vi "Get JTAG Scan Chain IDCODEs.vi"(8 "Error In":errorcluster, 11 "Adept Device":T1) -> (0 "Error In":errorcluster, 2 "IDCODEs":u32[](array[numeric]), 3 "Adept Device":T1)   [LabVIEW 2011, in "LVH-Adept.lvlib"]
doc: "Get the JTAG Scan Chain IDCODEs from a Digilent FPGA board."
uses:
  <vilib>/LabVIEW Hacker/Adept/LVH-Adept.lvlib
  Private/Type Defs/Device Config.ctl
  Private/Type Defs/Status.ctl
  Private/DJTG/DJTG.lvlib
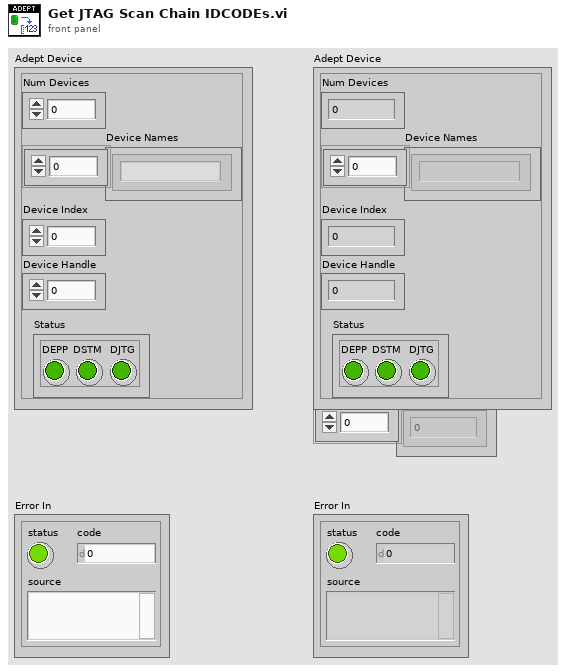
[diagram p1: front panel]
types:
  T1 = typedef "LVH-Adept.lvlib/Device Config.ctl" = cluster{"Num Devices":i32, "Device Names":string[], "Device Index":u16, "Device Handle":u32, "Status":T2}
  T2 = typedef "LVH-Adept.lvlib/Status.ctl" = cluster{"DEPP":bool, "DSTM":bool, "DJTG":bool}
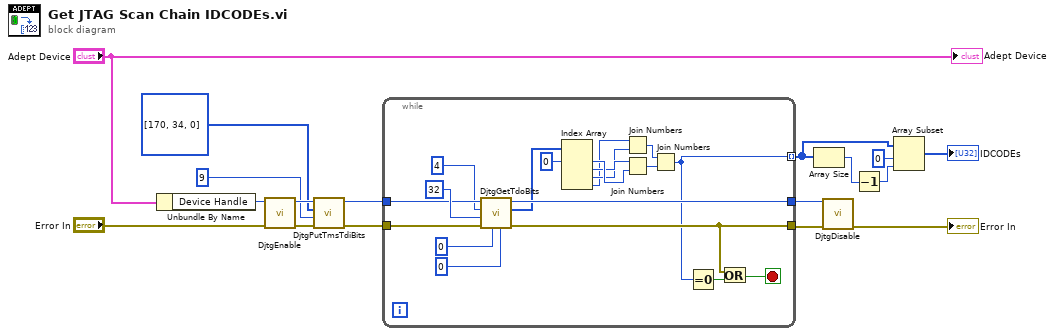
[diagram p0: block diagram]
diagram:
  n1 = Unbundle By Name("Adept Device") -> ("Device Handle"=w6:u32)
  n2 = call "DjtgEnable.vi"("Error In"="Error In", "Device Number"=w6) -> ("Error Out"=w17:errorcluster, "Device Number"=w16:u32)  [unwired: 8 in]
  n3 = call "DjtgPutTmsTdiBits.vi"("Error In"=w17, "Num Bit Pairs"=u32 9 ("cbitpairs"), "Data To Send"=u8[] [170, 34, 0] ("rgbSnd"), "Device Number"=w16) -> ("Error Out"=w13:errorcluster, "Device Number"=w12:u32)  [unwired: 5 in, 1 out]
  n4 = while {
    tunnel: w13 -> [w36]
    tunnel: w12 -> [w32]
    tunnel: [w31] -> w11
    tunnel: [w21] -> w10
    tunnel: [w20] -> w3 mode=indexing
    stop <- w19 stop-if-true
    n5 = call "DjtgGetTdoBits.vi"("TMS State"=u8 0 ("fTms"), "TDI State"=u8 0 ("fTdi"), "Error In"=w36, "Num Pit Pairs"=u32 32 ("cbitpairs"), "Data Buffer Size (bytes)"=4 ("rgbRec Buffer Size"), "Device Number"=w32) -> ("Error Out"=w21:errorcluster, "Data"=w30:u8[], "Device Number"=w31:u32)  [unwired: 3 in]
    n6 = Index Array(array=w30, index #1=0 ("index")) -> (element #1=w27:u8, element #2=w24:u8, element #3=w23:u8, element #4=w22:u8)  [unwired: 3 in]
    n7 = Join Numbers(hi=w22, lo=w23) -> ((hi.lo)=w25:u16)
    n8 = Join Numbers(hi=w24, lo=w27) -> ((hi.lo)=w26:u16)
    n9 = Join Numbers(hi=w25, lo=w26) -> ((hi.lo)=w20:u32)
    n10 = Equal To 0?(x=w20) -> (x = 0?=w18:bool)
    n11 = Or(x=w21, y=w18) -> (x .or. y?=w19:bool)
  }
  n12 = Array Size(array=w3) -> (size(s)=w2:i32)
  n13 = call "DjtgDisable.vi"("Error In"=w10, "Device Number"=w11) -> ("Error Out"=→"Error In":errorcluster)  [unwired: 8 in, 1 out]
  n14 = Decrement(x=w2) -> (x-1=w1:i32)
  n15 = Array Subset(array=w3, index=0, length=w1) -> (→"IDCODEs":u32[])
  "Adept Device" <- "Adept Device"
